vi "createModbusSubnetD.vi"(8 "error in (no error)":errorcluster, 11 "Boot in":refnum<class "Boot.lvclass">) -> (0 "error out":errorcluster, 2 "ModbusSubnetD":refnum<class "IModbus.lvclass">, 3 "Boot out":refnum<class "Boot.lvclass">)   [LabVIEW 2016, in "Boot.lvclass"]
uses:
  Boot.lvclass
  Common_RT_Modbus/IModbus/IModbus.lvclass
  Common_RT_Modbus/Modbus/Modbus.lvclass
  D:/Code/ts_M1M3Support/Common_RT_Modbus/IModbus/IModbus.lvclass
  Resources/ModbusSubnetDTxDataFIFO/ModbusSubnetDTxDataFIFO.lvclass
  D:/Code/ts_M1M3Support/Common_RT_FPGA/IWriteU16FIFO/IWriteU16FIFO.lvclass
  Boot.lvclass/Boot.ctl
  Resources/ModbusSubnetDTxDataFIFO/ModbusSubnetDTxDataFIFO.lvclass/ModbusSubnetDTxDataFIFO.ctl
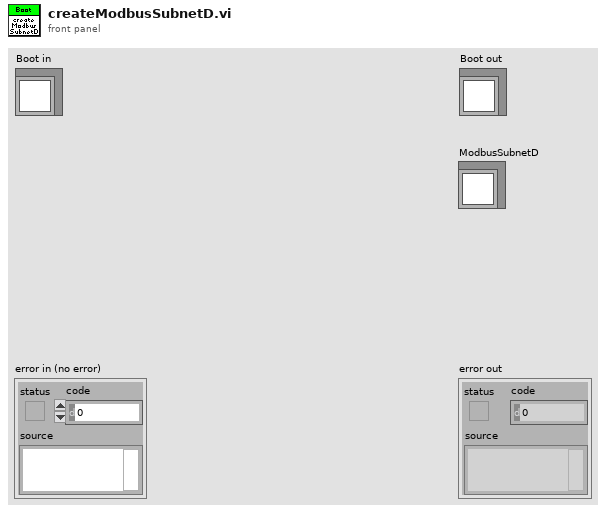
[diagram p1: front panel]
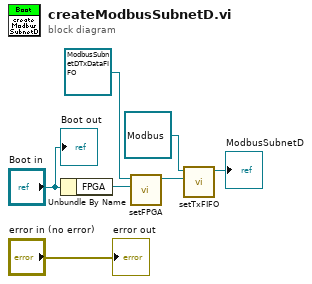
[diagram p0: block diagram]
diagram:
  n1 = Unbundle By Name("Boot in") -> ("FPGA"=w2:refnum<class "FPGA.lvclass">)
  n2 = call "setFPGA.vi"("FPGA"=w2, "ModbusSubnetDTxDataFIFO in"=refnum<class "ModbusSubnetDTxDataFIFO.lvclass"> refnum ("ModbusSubnetDTxDataFIFO.lvclass")) -> ("ModbusSubnetDTxDataFIFO out"=w1:refnum<class "ModbusSubnetDTxDataFIFO.lvclass">)  [unwired: 9 in]
  n3 = call "setTxFIFO.vi"("WriteU16FIFO"=w1, "Modbus in"=refnum<class "Modbus.lvclass"> refnum ("RTModbus.lvlib:Modbus.lvclass")) -> ("Modbus out"=→"ModbusSubnetD":refnum<class "Modbus.lvclass">)  [unwired: 9 in]
  "error out" <- "error in (no error)"
  "Boot out" <- "Boot in"
